vi "Initialize.vi"(8 "error in (no error)":errorcluster, 10 "Path":path=path "C:/Users/Albro/Downloads/Aditi_GDSII/Aditi_GDSII.gds", 11 "ParseGDSII in":refnum<class "ParseGDSII.lvclass">) -> (0 "error out":errorcluster, 3 "ParseGDSII out":refnum<class "ParseGDSII.lvclass">)   [LabVIEW 2019, in "ParseGDSII.lvclass"]
uses:
  ParseGDSII.lvclass
  ParseGDSII.lvclass/ParseGDSII.ctl
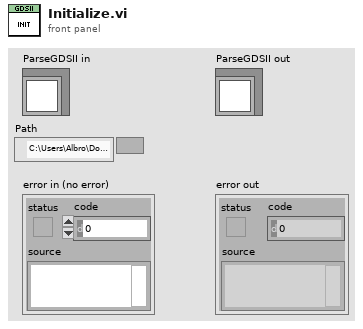
[diagram p1: front panel]
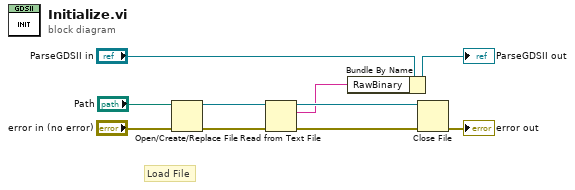
[diagram p0: block diagram]
diagram:
  # "Load File"
  n1 = Open/Create/Replace File(file path (use dialog)="Path", error in="error in (no error)") -> (refnum out=w9:refnum<file>, error out=w7:errorcluster)  [unwired: 4 in, 1 out]
  n2 = Read from Text File(file (use dialog)=w9, error in=w7) -> (refnum out=w8:refnum<file>, text=w3:string, error out=w6:errorcluster)  [unwired: 2 in, 1 out]
  n3 = Bundle By Name(cluster="ParseGDSII in", "RawBinary"=w3) -> (→"ParseGDSII out":refnum<class "ParseGDSII.lvclass">)
  n4 = Close File(refnum=w8, error in=w6) -> (error out=→"error out":errorcluster)  [unwired: 1 out]
